vi "Ensure Dependencies Created.vi"(5 "Owner Qualified Name":string, 8 "error in (no error)":errorcluster, 10 "Dependency Name":string, 11 "SMO in":refnum<class "SMO.lvclass">) -> (0 "error out":errorcluster, 2 "Unique Dependency name":string, 3 "SMO out":refnum<class "SMO.lvclass">)   [LabVIEW 2021, in "smo.lvlib" / "SMO.lvclass"]
uses:
  SMO.lvclass
  SMO.lvclass/SMO.ctl
  Support/Attribute.Identity/Attribute.Identity.lvclass/Attribute.Identity.ctl
  GetVariant(Attr).vi
  Support/Attribute.Identity/Read UniqueName.vi
  Support/Attribute.Identity/Read Given Name.vi
  Support/Attribute.Identity/Read ProspectiveOwner.vi
  ReftoDVR--SMO.vi
  Support/Attribute.Identity/Attribute.Identity.lvclass
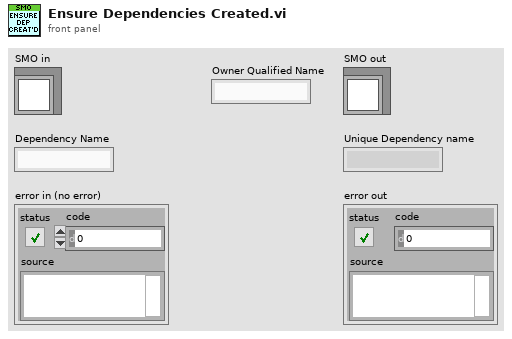
[diagram p1: front panel]
types:
  T1 = typedef "smo.lvlib/SMO.lvclass/SMOState --Enum.ctl" = enum16{"unknown", "Created", "Started", "Stopped"}
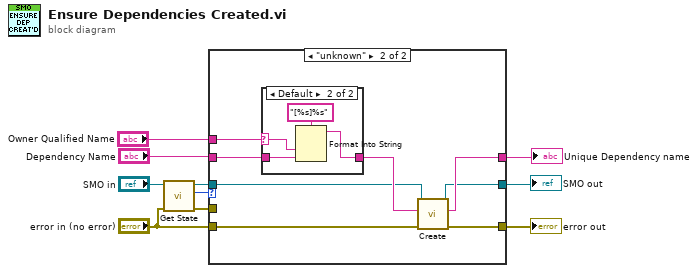
[diagram p0: block diagram]
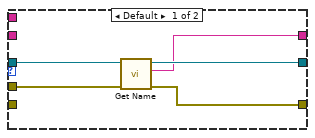
[diagram p2: hidden frame]
diagram:
  n1 = call "Get State.vi"("error in (no error)"="error in (no error)", "SMO"="SMO in") -> ("error out"=w6:errorcluster, "SMO State"=w7:T1, "SMO out"=w5:refnum<class "SMO.lvclass">)  [unwired: 7 in]
  n2 = case shown="\"unknown\"" w7 {
    tunnel: [w12 w18] -> w10
    tunnel: [w13 w16] -> w2
    tunnel: "Dependency Name" -> [_ w23]
    tunnel: [w11 w20] -> w9
    tunnel: w5 -> [w15 w17]
    tunnel: w6 -> [w14 _]
    tunnel: "error in (no error)" -> [_ w19]
    tunnel: "Owner Qualified Name" -> [_ w22]
    frame Default {
      n3 = call "Get Name.vi"("error in (no error)"=w14, "SMO"=w15) -> ("error out"=w12:errorcluster, "Name"=w11:string, "SMO out"=w13:refnum<class "SMO.lvclass">)  [unwired: 5 in, 2 out]
    }
    frame "unknown" {
      n4 = case shown="Default" w22 {
        selector: w22 -> [_ w25]
        tunnel: w23 -> [w24 w28]
        tunnel: [w24 w27] -> w21
        frame "" {
        }
        frame Default {
          n5 = Format Into String(format string="[%s]%s", w25, w28) -> (resulting string=w27:string)  [unwired: 2 in, 1 out]
        }
      }
      n6 = call "Create.vi"("error in (no error)"=w19, "Subsystem Name (optional)"=w21, "SMO"=w17) -> ("error out"=w18:errorcluster, "SMO name"=w20:string, "SMO out"=w16:refnum<class "SMO.lvclass">)  [unwired: 6 in]
    }
  }
  "error out" <- w10
  "Unique Dependency name" <- w9
  "SMO out" <- w2
